vi "zoom range.vi"(5 "zoom?":bool=TRUE, 7 "factor":dbl=1.0, 8 "window":dbl=0.01, 9 "center":dbl=0.01, 10 "left":dbl, 11 "right":dbl) -> (0 "window out":dbl, 1 "center out":dbl, 2 "left out":dbl, 3 "right out":dbl)   [LabVIEW 2015]
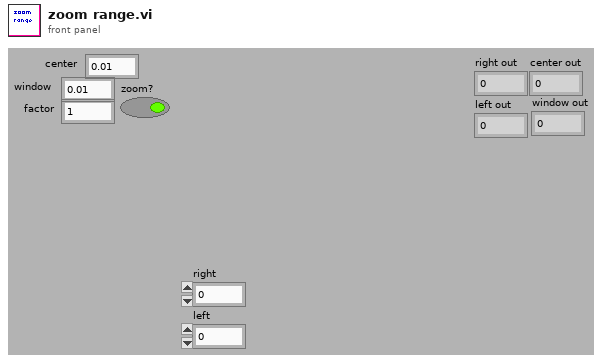
[diagram p1: front panel]
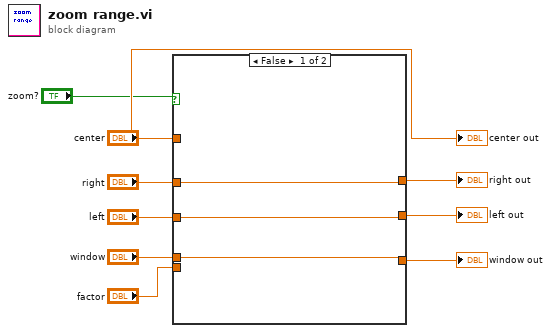
[diagram p0: block diagram]
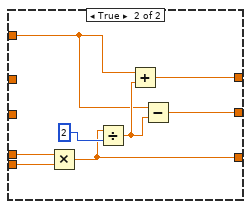
[diagram p2: hidden frame]
diagram:
  n1 = case shown="False" "zoom?" {
    tunnel: "window" -> [w10 w20]
    tunnel: "factor" -> [_ w19]
    tunnel: [w12 w16] -> w7
    tunnel: [w11 w15] -> w6
    tunnel: [w10 w14] -> w5
    tunnel: "center" -> [_ w13]
    tunnel: "right" -> [w12 _]
    tunnel: "left" -> [w11 _]
    frame False {
    }
    frame True {
      n2 = Multiply(x=w20, y=w19) -> (x*y=w14:dbl)
      n3 = Divide(x=w14, y=2) -> (x/y=w17:dbl)
      n4 = Add(x=w13, y=w17) -> (x+y=w16:dbl)
      n5 = Subtract(x=w13, y=w17) -> (x-y=w15:dbl)
    }
  }
  "right out" <- w7
  "left out" <- w6
  "window out" <- w5
  "center out" <- "center"
